vi "Trajectory_TransformBy.vi"(9 "TRANSFORM":T6={"TRANSLATION"={"X"=0.0, "Y"=0.0}, "ROTATION"={"VALUE"=0.0, "COS"=1.0, "SIN"=0.0}} {"ROTATION"."SIN" format="%13.4f"; "ROTATION"."COS" format="%13.4f"; "ROTATION"."VALUE" format="%13.4f"; "TRANSLATION"."Y" format="%14.3f"; "TRANSLATION"."X" format="%14.3f"}, 11 "InputTRAJECTORY":T1 {"States"."POSE"."ROTATION"."SIN" format="%13.4f"; "States"."POSE"."ROTATION"."COS" format="%13.4f"; "States"."POSE"."ROTATION"."VALUE" format="%13.4f"; "States"."POSE"."TRANSLATION"."Y" format="%14.3f"; "States"."POSE"."TRANSLATION"."X" format="%14.3f"; "TotalTImeSecs" format="%20.3f"}) -> (3 "outputTRAJECTORY":T1 {"States"."POSE"."ROTATION"."SIN" format="%13.4f"; "States"."POSE"."ROTATION"."COS" format="%13.4f"; "States"."POSE"."ROTATION"."VALUE" format="%13.4f"; "States"."POSE"."TRANSLATION"."Y" format="%14.3f"; "States"."POSE"."TRANSLATION"."X" format="%14.3f"; "TotalTImeSecs" format="%20.3f"})   [LabVIEW 2019, in "Trajectory_Library.lvlib"]
doc: "Transforms all poses in the trajectory by the given transform. This is useful for converting a robot-relative trajectory into a field-relative trajectory. This works with respect to the first pose in the trajectory.\n \nParameters:\n - InputTrajectory - Trajectory data structure\n - transform - The transform to transform the trajectory by.\n\nReturns:\n - OutputTrajectory - The transformed trajectory."
uses:
  Trajectory_Library.lvlib
  TRAJECTORY.ctl
  TRAJ_STATE.ctl
  POSE2D.ctl
  TRANSLATION2D.ctl
  ROTATION2D.ctl
  TRANSFORM2D.ctl
  Pose_TransformBy.vi
  Pose_RelativeTo.vi
  Transform_Create_TransRot.vi
  Translation_RotateBy.vi
  Translation_Plus.vi
  Rotation_Plus.vi
  Pose_New_TRRO.vi
  Transform_Create_PosePose.vi
  Translation_Create.vi
  Rotation_RotateBy.vi
  Rotation_UnaryMinus.vi
  Translation_Minus.vi
  Rotation_Minus.vi
  Rotation_CreateXY.vi
  Rotation_CreateAngle.vi
  Util_CalcDist.vi
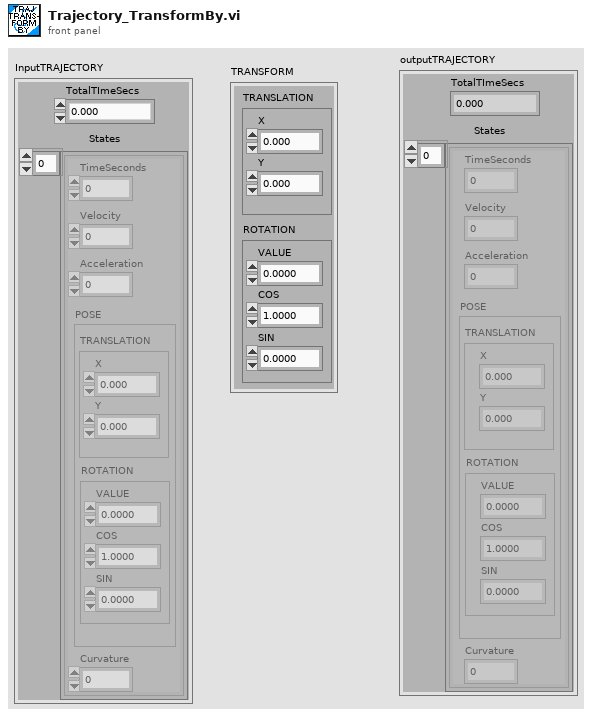
[diagram p1: front panel]
types:
  T1 = typedef "Trajectory_Library.lvlib/TRAJECTORY.ctl" = cluster{"TotalTImeSecs":dbl, "States":T2[]}
  T2 = typedef "Trajectory_Library.lvlib/TRAJ_STATE.ctl" = cluster{"TimeSeconds":dbl, "Velocity":dbl, "Acceleration":dbl, "POSE":T3, "Curvature":dbl}
  T3 = typedef "Trajectory_Library.lvlib/POSE2D.ctl" = cluster{"TRANSLATION":T4, "ROTATION":T5}
  T4 = typedef "Trajectory_Library.lvlib/TRANSLATION2D.ctl" = cluster{"X":dbl, "Y":dbl}
  T5 = typedef "Trajectory_Library.lvlib/ROTATION2D.ctl" = cluster{"VALUE":dbl, "COS":dbl, "SIN":dbl}
  T6 = typedef "Trajectory_Library.lvlib/TRANSFORM2D.ctl" = cluster{"TRANSLATION":T4, "ROTATION":T5}
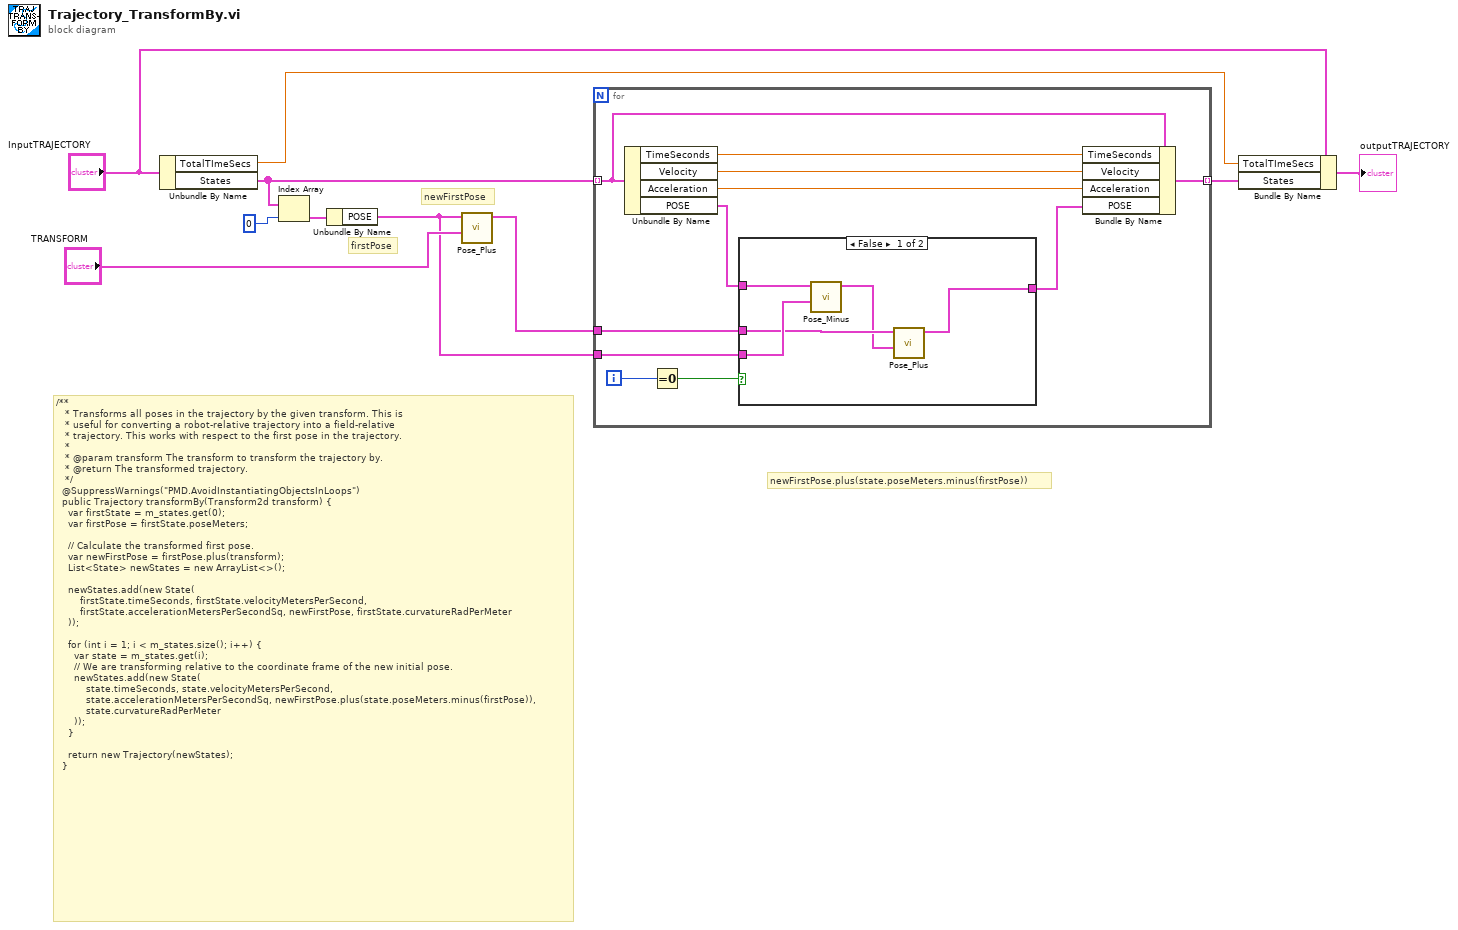
[diagram p0: block diagram]
diagram:
  # "newFirstPose"
  # "firstPose"
  # "newFirstPose.plus(state.poseMeters.minus(firstPose))"
  # "/**\n   * Transforms all poses in the trajectory by the given transform. This is\n   * useful for converting a robot-relative trajectory into a field-relative\n   * trajectory. This works with respect to the first pose in the trajectory.\n   *\n   * @param transform The transform to transform the trajectory by.\n   * @return The transformed trajectory.\n   */\n  @SuppressWarnings(\"PMD.AvoidInstantiatingObjectsInLoops\")\n  public Trajectory transformBy(Transform2d transform) {\n    var firstState = m_states.get(0);\n    var firstPose = firstState.poseMeters;\n\n    // Calculate the transformed first pose.\n    var newFirstPose = firstPose.plus(transform);\n    List<State> newStates = new ArrayList<>();\n\n    newStates.add(new State(\n        firstState.timeSeconds, firstState.velocityMetersPerSecond,\n        firstState.accelerationMetersPerSecondSq, newFirstPose, firstState.curvatureRadPerMeter\n    ));\n\n    for (int i = 1; i < m_states.size(); i++) {\n      var state = m_states.get(i);\n      // We are transforming relative to the coordinate frame of the new initial pose.\n      newStates.add(new State(\n          state.timeSeconds, state.velocityMetersPerSecond,\n          state.accelerationMetersPerSecondSq, newFirstPose.plus(state.poseMeters.minus(firstPose)),\n          state.curvatureRadPerMeter\n      ));\n    }\n\n    return new Trajectory(newStates);\n  }"
  n1 = Unbundle By Name("InputTRAJECTORY") -> ("TotalTImeSecs"=w9:dbl, "States"=w6:T2[])
  n2 = Index Array(array=w6, index=0) -> (element=w4:T2)
  n3 = Unbundle By Name(w4) -> ("POSE"=w1:T3)
  n4 = call "Pose_Plus.vi"("other TRANSFORM"="TRANSFORM", "in POSE"=w1) -> ("out POSE"=w2:T3)  [unwired: 9 in]
  n5 = for {
    tunnel: w6 -> [w21] mode=indexing
    tunnel: [w20] -> w8 mode=indexing
    tunnel: w2 -> [w14]
    tunnel: w1 -> [w11]
    i -> [w16]
    n6 = Unbundle By Name(w21) -> ("TimeSeconds"=w19:dbl, "Velocity"=w18:dbl, "Acceleration"=w17:dbl, "POSE"=w12:T3)
    n7 = Equal To 0?(x=w16) -> (x = 0?=w15:bool)
    n8 = case shown="False" w15 {
      tunnel: [w22 w27] -> w13
      tunnel: w14 -> [w24 w27]
      tunnel: w12 -> [w26 _]
      tunnel: w11 -> [w25 _]
      frame False {
        n9 = call "Pose_Minus.vi"("other TRANSFORM"=w25, "in POSE"=w26) -> ("outTRANSFORM"=w23:T6)  [unwired: 9 in]
        n10 = call "Pose_Plus.vi"("other TRANSFORM"=w23, "in POSE"=w24) -> ("out POSE"=w22:T3)  [unwired: 9 in]
      }
      frame True {
      }
    }
    n11 = Bundle By Name(cluster=w21, "TimeSeconds"=w19, "Velocity"=w18, "Acceleration"=w17, "POSE"=w13) -> (w20:T2)
  }
  n12 = Bundle By Name(cluster="InputTRAJECTORY", "TotalTImeSecs"=w9, "States"=w8) -> (→"outputTRAJECTORY":T1)
